vi "ModemTelemetryParser.vi"(7 "Operation":enum16{"Parse", "Initialize"}(ring), 8 "Error In":errorcluster, 9 "Frame Size":i32=32, 11 "Serial Data In":string) -> (0 "Error Out":errorcluster, 3 "Detected Frames":u8[][](array[numeric]))   [LabVIEW 2010]
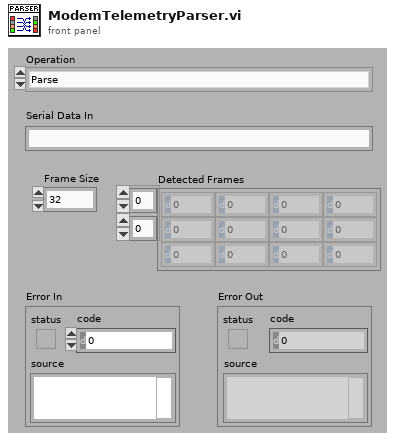
[diagram p1: front panel]
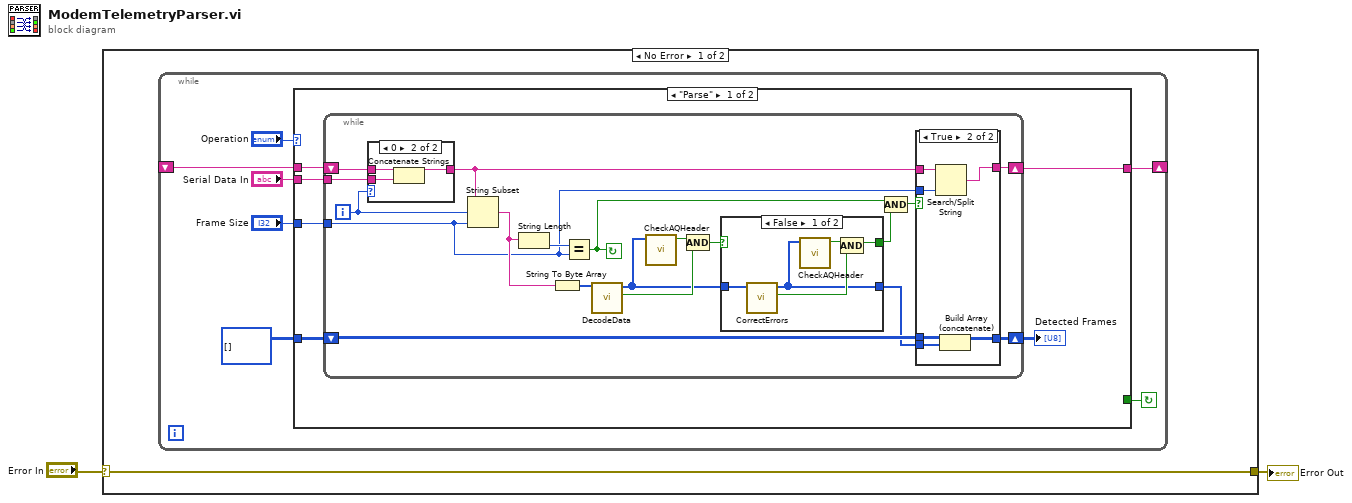
[diagram p0: block diagram]
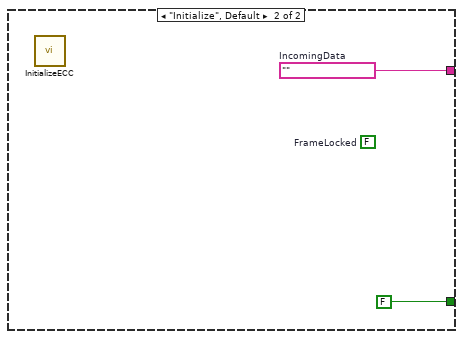
[diagram p5: hidden frame]
diagram:
  n1 = case shown="No Error" "Error In" {
    selector: "Error In" -> [w3 w57]
    tunnel: [w3 w57] -> w1
    frame No Error {
      n2 = while {
        shift-right: [w9] -> _
        shift-left: _ -> [w8]
        stop <- w5 continue-if-true
        n3 = case shown="\"Parse\"" "Operation" {
          tunnel: [w14 w56] -> w9
          tunnel: w8 -> [w16 _]
          tunnel: "Serial Data In" -> [w15 _]
          tunnel: "Frame Size" -> [w13 _]
          tunnel: [_ FALSE] -> w5
          tunnel: u8[][] [] ("Encoded Data Out") -> [w12 _]
          frame "Parse" {
            n4 = while {
              shift-right: [w23] -> w14
              shift-left: w16 -> [w35]
              tunnel: w15 -> [w34]
              tunnel: w13 -> [w24]
              shift-right: [w17] -> w11
              shift-left: w12 -> [w19]
              i -> [w33]
              stop <- w20 continue-if-true
              n5 = case shown="0" w33 {
                tunnel: w35 -> [w51 w54]
                tunnel: w34 -> [_ w53]
                tunnel: [w51 w52] -> w25
                frame Default {
                }
                frame 0 {
                  n6 = Concatenate Strings(w54, w53) -> (w52:string)
                }
              }
              n7 = String Subset(string=w25, offset (0)=w33, length (rest)=w24) -> (substring=w26:string)
              n8 = String Length(string=w26) -> (length=w32:i32)
              n9 = String To Byte Array(string=w26) -> (unsigned byte array=w31:u8[])
              n10 = Equal?(x=w32, y=w24) -> (x = y?=w20:bool)
              n11 = call "DecodeData.vi"("Encoded Data"=w31) -> ("Check Syndrome"=w30:bool, "Encoded Data Out"=w28:u8[])  [unwired: 8 in, 1 out]
              n12 = call "CheckAQHeader.vi"("Encoded Data In"=w28) -> ("Header Found"=w29:bool)  [unwired: 9 in, 1 out]
              n13 = Compound Arithmetic op=AND(w29, w30) -> (w27:bool)
              n14 = case shown="False" w27 {
                selector: w27 -> [_ w50]
                tunnel: w28 -> [w48 w49]
                tunnel: [w45 w50] -> w22
                tunnel: [w44 w49] -> w18
                frame False {
                  n15 = call "CorrectErrors.vi"("Encoded Data"=w48) -> ("Success"=w46:bool, "Corrected Data"=w44:u8[])  [unwired: 8 in, 1 out]
                  n16 = call "CheckAQHeader.vi"("Encoded Data In"=w44) -> ("Header Found"=w47:bool)  [unwired: 9 in, 1 out]
                  n17 = Compound Arithmetic op=AND(w47, w46) -> (w45:bool)
                }
                frame True {
                }
              }
              n18 = Compound Arithmetic op=AND(w20, w22) -> (w21:bool)
              n19 = case shown="True" w21 {
                tunnel: w25 -> [w37 w43]
                tunnel: w24 -> [_ w42]
                tunnel: [w37 w41] -> w23
                tunnel: w19 -> [w36 w40]
                tunnel: w18 -> [_ w39]
                tunnel: [w36 w38] -> w17
                frame False {
                }
                frame True {
                  n20 = Search/Split String(string=w43, offset (0)=w42) -> (match + rest of string=w41:string)  [unwired: 1 in, 2 out]
                  n21 = Build Array (concatenate)(w40, w39) -> (w38:u8[][])
                }
              }
            }
            "Detected Frames" <- w11
          }
          frame "Initialize", Default {
            (unwired) FALSE  # FrameLocked
            w56 = ""  # IncomingData
            n22 = call "InitializeECC.vi"() -> ()  [unwired: 11 in, 1 out]
          }
        }
      }
    }
    frame Error {
    }
  }
  "Error Out" <- w1
